vi "Grab.vi"() -> (0 "rollers":dbl, 3 "shoulder":dbl)   [LabVIEW 2014]
uses:
  Events.vi
  <vilib>/ptbypt/NI_PtbyPt.lvlib
panel:
  out "At point":bool
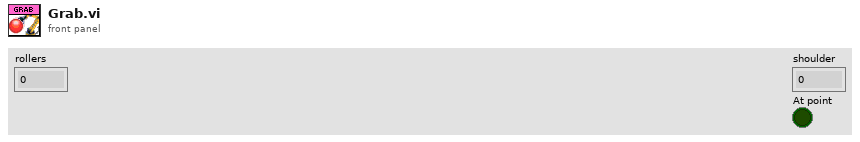
[diagram p1: front panel]
types:
  T1 = typedef "Eventgrab.ctl" = cluster{"Grab":bool, "GroundPass":bool, "Test Aqaure":dbl, "Shoulder up or down?":bool, "Auton drag":bool}
  T2 = typedef "WPI_SolenoidValue.ctl" = enum16{"Off", "On", "Forward", "Reverse"}
  T3 = cluster{"Ultrasonic Distance (In)":dbl, "Gyro":dbl, "TopAquisition sensor":bool, "Encoder distance":dbl, "Encoder rate":dbl, "Encoder direction":bool, "winch engaged?":T2, "Motor Values":dbl[], "Latch encoder":u32, "BottomAquistion":bool, "BottomAquistion 2":bool, "Gyro Rate":dbl}
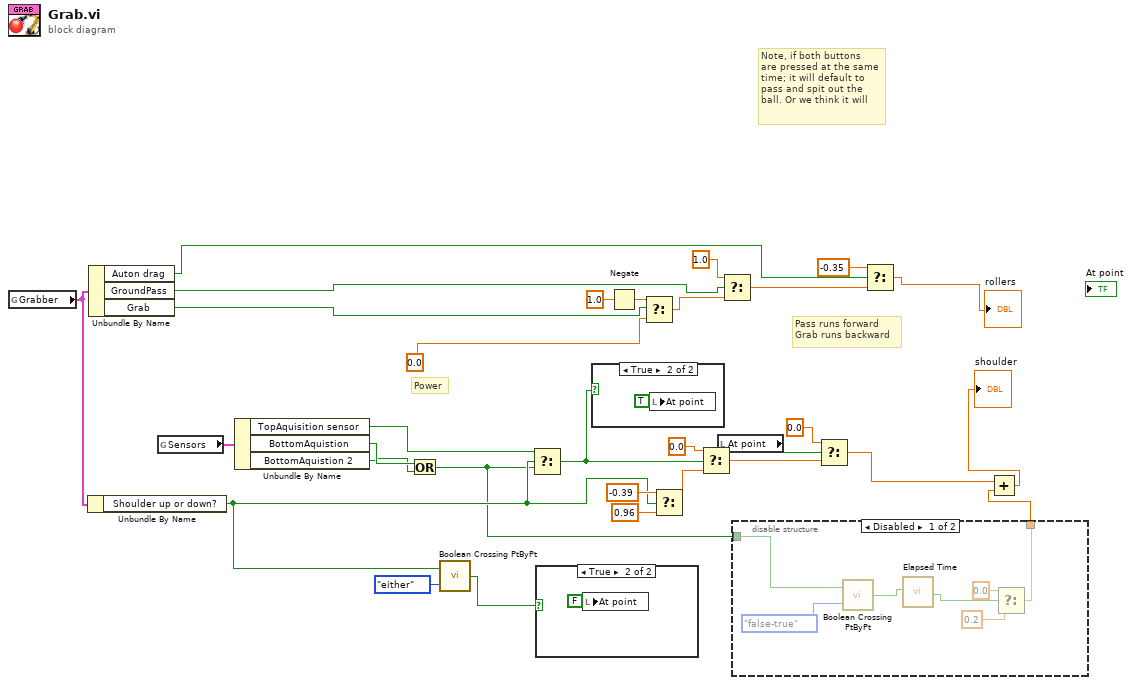
[diagram p0: block diagram]
diagram:
  # "Pass runs forward\nGrab runs backward"
  # "Note, if both buttons\nare pressed at the same\ntime; it will default to\npass and spit out the\nball. Or we think it will"
  # "Power"
  n1 = global read "Events.vi" "Grabber"() -> (w24:T1)
  n2 = Unbundle By Name(w24) -> ("Shoulder up or down?"=w9:bool)
  n3 = Unbundle By Name(w24) -> ("Auton drag"=w2:bool, "GroundPass"=w27:bool, "Grab"=w28:bool)
  n4 = global read "Events.vi" "Sensors"() -> (w19:T3)
  n5 = Unbundle By Name(w19) -> ("TopAquisition sensor"=w18:bool, "BottomAquistion"=w11:bool, "BottomAquistion 2"=w10:bool)
  n6 = Or(x=w11, y=w10) -> (x .or. y?=w8:bool)
  n7 = call <vilib>:"Boolean Crossing PtByPt.vi"("direction"=enum16{"either", "false-true", "true-false"}."either", "input"=w9) -> ("crossing"=w13:bool)  [unwired: 1 in]
  n8 = Select(t=w18, s=w9, f=w8) -> (s? t:f=w15:bool)
  n9 = case shown="True" w13 {
    frame False {
    }
    frame True {
      n10 = local write "At point"(FALSE ("s? t:f")) -> ()
    }
  }
  n11 = case shown="True" w15 {
    frame False {
    }
    frame True {
      n12 = local write "At point"(TRUE ("s? t:f")) -> ()
    }
  }
  n13 = Negate(x=1.0 ("Power")) -> (-x=w29:dbl)
  n14 = Select(t=w29, s=w28, f=0.0) -> (s? t:f=w30:dbl)
  n15 = Select(t=-0.39, s=w9, f=0.96) -> (s? t:f=w20:dbl)
  n16 = Select(t=0.0, s=w15, f=w20) -> (s? t:f=w17:dbl)
  n17 = local read "At point"() -> (w14:bool)
  n18 = Select(t=1.0, s=w27, f=w30) -> (s? t:f=w4:dbl)
  n19 = disable-structure shown="Disabled" {
    disable-tunnel: w8 -> [w39 _]
    disable-tunnel: [w34 _] -> w7
    frame Disabled {
      n20 = call <vilib>:"Boolean Crossing PtByPt.vi"("direction"=enum16{"either", "false-true", "true-false"}."false-true", "input"=w39) -> ("crossing"=w38:bool)  [unwired: 1 in]
      n21 = call "Elapsed Time"("Reset"=w38) -> ("Time has Elapsed"=w37:bool)  [unwired: 11 in, 7 out]
      n22 = Select(t=0.0, s=w37, f=0.2) -> (s? t:f=w34:dbl)
    }
    frame Enabled {
    }
  }
  n23 = Select(t=0.0, s=w14, f=w17) -> (s? t:f=w6:dbl)
  n24 = Select(t=-0.35, s=w2, f=w4) -> (s? t:f=→"rollers":dbl)
  n25 = Add(x=w6, y=w7) -> (x+y=→"shoulder":dbl)
